vi "Test Timer.vi"() -> ()   [LabVIEW 2012]
doc: "This is an example of how to use the Output Timer class to control the switching behavior fo the CAT system."
uses:
  MSE CAT Controller Demo Source/Type Defs/Output Values.ctl
  MSE CAT Controller Demo Source/Type Defs/AD Settings.ctl
  MSE CAT Controller Demo Source/Type Defs/Output Switches.ctl
  Output Timer/Output Timer.lvclass
  Output Timer/Output Timer.lvclass/Output Timer.ctl
panel:
  out "Numeric":i32
  out "Last Switch":T1 {"[0]" format="%<%H:%M:%S%2u>T"; "[1]" format="%<%H:%M:%S%2u>T"; "[2]" format="%<%H:%M:%S%2u>T"; "[3]" format="%<%H:%M:%S%2u>T"; "[4]" format="%<%H:%M:%S%2u>T"; "[5]" format="%<%H:%M:%S%2u>T"; "[6]" format="%<%H:%M:%S%2u>T"; "[7]" format="%<%H:%M:%S%2u>T"; "[8]" format="%<%H:%M:%S%2u>T"; "[9]" format="%<%H:%M:%S%2u>T"; "[10]" format="%<%H:%M:%S%2u>T"; "[11]" format="%<%H:%M:%S%2u>T"; "[12]" format="%<%H:%M:%S%2u>T"; "[13]" format="%<%H:%M:%S%2u>T"; "[14]" format="%<%H:%M:%S%2u>T"; "[15]" format="%<%H:%M:%S%2u>T"; "[16]" format="%<%H:%M:%S%2u>T"; "[17]" format="%<%H:%M:%S%2u>T"; "[18]" format="%<%H:%M:%S%2u>T"; "[19]" format="%<%H:%M:%S%2u>T"; "[20]" format="%<%H:%M:%S%2u>T"}
  out "Time Stamp":timestamp format="%<%H:%M:%S%2u>T"
  out "Delay S":T2={"Main 1"=inf, "Main 2"=inf, "Recirc  3"=9000.0, "Scrub 4"=8800.0, "O2 5"=9600.0, "Vent 6"=9200.0, "Boost A 7"=3400.0, "Boost A 8"=3400.0, "Recirc  9"=9000.0, "Scrub 10"=8800.0, "Vent 11"=9200.0, "Boost B 12"=1800.0, "Boost B 13"=1800.0, "Recirc 14"=9000.0, "Scrub 15"=8800.0, "Vent 16"=9200.0, "Main 17"=inf, "Boost A 18"=3400.0, "Boost B 19"=1800.0, "Boost F 20"=7000.0, "Vent 2 21"=9200.0}
  out "Final Out":T3
  in  "Final In":T3
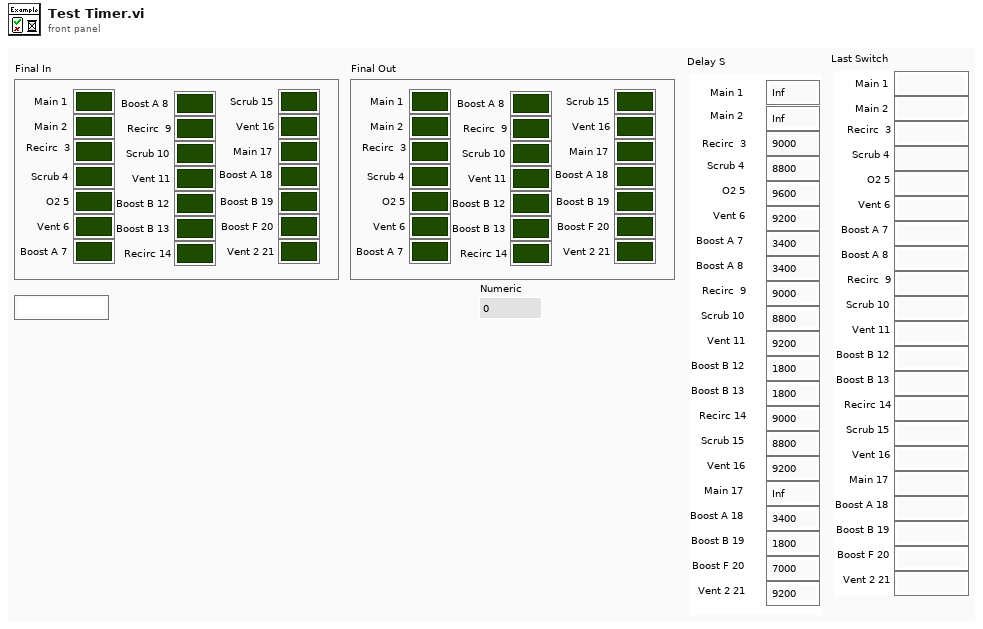
[diagram p1: front panel]
types:
  T1 = cluster{"[0]":timestamp, "[1]":timestamp, "[2]":timestamp, "[3]":timestamp, "[4]":timestamp, "[5]":timestamp, "[6]":timestamp, "[7]":timestamp, "[8]":timestamp, "[9]":timestamp, "[10]":timestamp, "[11]":timestamp, "[12]":timestamp, "[13]":timestamp, "[14]":timestamp, "[15]":timestamp, "[16]":timestamp, "[17]":timestamp, "[18]":timestamp, "[19]":timestamp, "[20]":timestamp}
  T2 = typedef "Output Values.ctl" = cluster{"Main 1":dbl, "Main 2":dbl, "Recirc  3":dbl, "Scrub 4":dbl, "O2 5":dbl, "Vent 6":dbl, "Boost A 7":dbl, "Boost A 8":dbl, "Recirc  9":dbl, "Scrub 10":dbl, "Vent 11":dbl, "Boost B 12":dbl, "Boost B 13":dbl, "Recirc 14":dbl, "Scrub 15":dbl, "Vent 16":dbl, "Main 17":dbl, "Boost A 18":dbl, "Boost B 19":dbl, "Boost F 20":dbl, "Vent 2 21":dbl}
  T3 = cluster{"Main 1":bool, "Main 2":bool, "Recirc  3":bool, "Scrub 4":bool, "O2 5":bool, "Vent 6":bool, "Boost A 7":bool, "Boost A 8":bool, "Recirc  9":bool, "Scrub 10":bool, "Vent 11":bool, "Boost B 12":bool, "Boost B 13":bool, "Recirc 14":bool, "Scrub 15":bool, "Vent 16":bool, "Main 17":bool, "Boost A 18":bool, "Boost B 19":bool, "Boost F 20":bool, "Vent 2 21":bool}
  T4 = typedef "AD Settings.ctl" = cluster{"Set Point Force":T2, "Run A1":T2, "Run A2":T2, "Hold A3":T2, "Hold A4":T2, "High AD Diff ":T5, "Delay S":T2}
  T5 = typedef "Output Switches.ctl" = cluster{"Main 1":bool, "Main 2":bool, "Recirc  3":bool, "Scrub 4":bool, "O2 5":bool, "Vent 6":bool, "Boost A 7":bool, "Boost A 8":bool, "Recirc  9":bool, "Scrub 10":bool, "Vent 11":bool, "Boost B 12":bool, "Boost B 13":bool, "Recirc 14":bool, "Scrub 15":bool, "Vent 16":bool, "Main 17":bool, "Boost A 18":bool, "Boost B 19":bool, "Boost F 20":bool, "Vent 2 21":bool}
  T6 = cluster{"[0]":bool, "[1]":bool, "[2]":bool, "[3]":bool, "[4]":bool, "[5]":bool, "[6]":bool, "[7]":bool, "[8]":bool, "[9]":bool, "[10]":bool, "[11]":bool, "[12]":bool, "[13]":bool, "[14]":bool, "[15]":bool, "[16]":bool, "[17]":bool, "[18]":bool, "[19]":bool, "[20]":bool}
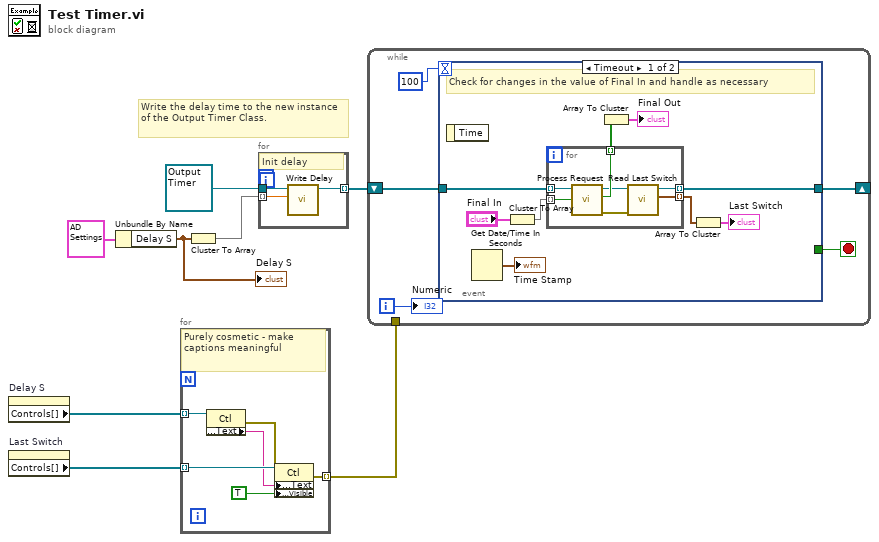
[diagram p0: block diagram]
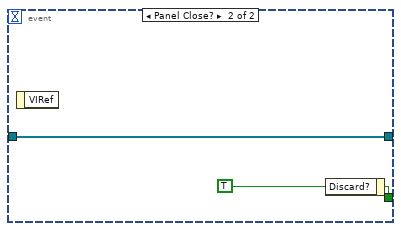
[diagram p2: hidden frame]
diagram:
  # "Write the delay time to the new instance of the Output Timer Class."
  n1 = property on="Delay S" class="Clust (strict)"() -> ("Controls[]"=w3:refnum<vi>[])  [unwired: 2 in, 2 out]
  n2 = property on="Last Switch" class="Clust (strict)"() -> ("Controls[]"=w2:refnum<vi>[])  [unwired: 2 in, 2 out]
  n3 = Unbundle By Name(T4 {"Set Point Force"={"Main 1"=inf, "Main 2"=inf, "Recirc  3"=inf, "Scrub 4"=inf, "O2 5"=inf, "Vent 6"=inf, "Boost A 7"=inf, "Boost A 8"=inf, "Recirc  9"=inf, "Scrub 10"=inf, "Vent 11"=inf, "Boost B 12"=inf, "Boost B 13"=inf, "Recirc 14"=inf, "Scrub 15"=inf, "Vent 16"=inf, "Main 17"=inf, "Boost A 18"=inf, "Boost B 19"=inf, "Boost F 20"=6000.0, "Vent 2 21"=inf}, "Run A1"={"Main 1"=inf, "Main 2"=inf, "Recirc  3"=50.0, "Scrub 4"=inf, "O2 5"=150.0, "Vent 6"=60.0, "Boost A 7"=0.0, "Boost A 8"=0.0, "Recirc  9"=50.0, "Scrub 10"=inf, "Vent 11"=60.0, "Boost B 12"=15.0, "Boost B 13"=15.0, "Recirc 14"=50.0, "Scrub 15"=inf, "Vent 16"=60.0, "Main 17"=inf, "Boost A 18"=0.0, "Boost B 19"=15.0, "Boost F 20"=0.0, "Vent 2 21"=700.0}, "Run A2"={"Main 1"=inf, "Main 2"=inf, "Recirc  3"=-30.0, "Scrub 4"=inf, "O2 5"=80.0, "Vent 6"=15.0, "Boost A 7"=-80.0, "Boost A 8"=-80.0, "Recirc  9"=-30.0, "Scrub 10"=inf, "Vent 11"=15.0, "Boost B 12"=-50.0, "Boost B 13"=-50.0, "Recirc 14"=-30.0, "Scrub 15"=inf, "Vent 16"=15.0, "Main 17"=inf, "Boost A 18"=0.0, "Boost B 19"=-50.0, "Boost F 20"=-80.0, "Vent 2 21"=650.0}, "Hold A3"={"Main 1"=0.0, "Main 2"=0.0, "Recirc  3"=50.0, "Scrub 4"=inf, "O2 5"=150.0, "Vent 6"=60.0, "Boost A 7"=-150.0, "Boost A 8"=-150.0, "Recirc  9"=50.0, "Scrub 10"=inf, "Vent 11"=60.0, "Boost B 12"=-200.0, "Boost B 13"=-200.0, "Recirc 14"=50.0, "Scrub 15"=inf, "Vent 16"=60.0, "Main 17"=0.0, "Boost A 18"=-150.0, "Boost B 19"=-200.0, "Boost F 20"=-200.0, "Vent 2 21"=650.0}, "Hold A4"={"Main 1"=-150.0, "Main 2"=-150.0, "Recirc  3"=-30.0, "Scrub 4"=inf, "O2 5"=80.0, "Vent 6"=15.0, "Boost A 7"=-250.0, "Boost A 8"=-250.0, "Recirc  9"=-30.0, "Scrub 10"=inf, "Vent 11"=15.0, "Boost B 12"=-300.0, "Boost B 13"=-300.0, "Recirc 14"=-30.0, "Scrub 15"=inf, "Vent 16"=15.0, "Main 17"=-150.0, "Boost A 18"=-250.0, "Boost B 19"=-300.0, "Boost F 20"=-300.0, "Vent 2 21"=650.0}, "High AD Diff "={"Main 1"=FALSE, "Main 2"=FALSE, "Recirc  3"=FALSE, "Scrub 4"=TRUE, "O2 5"=FALSE, "Vent 6"=TRUE, "Boost A 7"=FALSE, "Boost A 8"=FALSE, "Recirc  9"=FALSE, "Scrub 10"=TRUE, "Vent 11"=TRUE, "Boost B 12"=FALSE, "Boost B 13"=FALSE, "Recirc 14"=FALSE, "Scrub 15"=TRUE, "Vent 16"=TRUE, "Main 17"=FALSE, "Boost A 18"=FALSE, "Boost B 19"=FALSE, "Boost F 20"=FALSE, "Vent 2 21"=TRUE}, "Delay S"={"Main 1"=30.0, "Main 2"=30.0, "Recirc  3"=1.0, "Scrub 4"=1.0, "O2 5"=1.0, "Vent 6"=1.0, "Boost A 7"=30.0, "Boost A 8"=30.0, "Recirc  9"=1.0, "Scrub 10"=1.0, "Vent 11"=1.0, "Boost B 12"=30.0, "Boost B 13"=30.0, "Recirc 14"=1.0, "Scrub 15"=1.0, "Vent 16"=1.0, "Main 17"=30.0, "Boost A 18"=30.0, "Boost B 19"=30.0, "Boost F 20"=30.0, "Vent 2 21"=1.0}} ("AD Settings")) -> ("Delay S"=w8:T2)
  "Delay S" <- w8
  n4 = for {
    tunnel: w3 -> [w14] mode=indexing
    tunnel: w2 -> [w13] mode=indexing
    tunnel: [w10] -> w1 mode=indexing
    # "Purely cosmetic - make captions meaningful"
    n5 = property class="Ctl"(reference=w14) -> (error out=w11:errorcluster, "Label.Text"=w12:string)  [unwired: 1 in, 1 out]
    n6 = property class="Ctl"(reference=w13, error in=w11, "Caption.Text"=w12, "Caption.Visible"=TRUE) -> (error out=w10:errorcluster)  [unwired: 1 out]
  }
  n7 = Cluster To Array(cluster=w8) -> (array=w7:dbl[])
  n8 = for {
    tunnel: w7 -> [w16] mode=indexing
    tunnel: refnum<class "Output Timer.lvclass"> refnum ("Delay Timer") -> [w17]
    tunnel: [w15] -> w4 mode=indexing
    # "Init delay"
    n9 = call "Write Delay.vi"("Delay"=w16, "Output Timer in"=w17) -> ("Output Timer out"=w15:refnum<class "Output Timer.lvclass">)  [unwired: 8 in, 1 out]
  }
  n10 = while {
    shift-right: [w21] -> _
    shift-left: w4 -> [w22]
    tunnel: w1 -> [_]
    i -> [w18]
    stop <- w19 stop-if-true
    n11 = event shown="[0] Timeout" {
      selector: _ -> [_ _]
      dyn-events: _ -> [_ _]
      timeout: 100 ("Period") -> [_ _]
      tunnel: w22 -> [w29 w39]
      tunnel: [w28 w39] -> w21
      tunnel: [_ w40] -> w19
      event Timeout {
        # "Check for changes in the value of Final In and handle as necessary"
        n12 = event-data() -> ()  [unwired: 1 in, 1 out]
        n13 = Get Date/Time In Seconds() -> (seconds since 1Jan1904=→"Time Stamp":timestamp)
        n14 = Cluster To Array(cluster="Final In") -> (array=w30:bool[])
        n15 = for {
          tunnel: w29 -> [w38] mode=indexing
          tunnel: w30 -> [w37] mode=indexing
          tunnel: [w33] -> w28 mode=indexing
          tunnel: [w36] -> w27 mode=indexing
          tunnel: [w32] -> w24 mode=indexing
          n16 = call "Process Request.vi"("Requested"=w37, "Delay Timer in"=w38) -> ("error out"=w34:errorcluster, "Returned"=w36:bool, "Delay Timer out"=w35:refnum<class "Output Timer.lvclass">)  [unwired: 7 in]
          n17 = call "Read Last Switch.vi"("error in (no error)"=w34, "Output Timer in"=w35) -> ("Last Switch"=w32:timestamp, "Output Timer out"=w33:refnum<class "Output Timer.lvclass">)  [unwired: 7 in, 1 out]
        }
        n18 = Array To Cluster(array=w27) -> (cluster=→"Final Out":T6)
        n19 = Array To Cluster(array=w24) -> (cluster=→"Last Switch":T1)
      }
      event Panel Close? {
        w40 = TRUE ("Discard?")
        n20 = event-data() -> ()  [unwired: 1 in, 1 out]
        n21 = event-data("Discard?"=w40) -> ()  [unwired: 1 in, 1 out]
      }
    }
    "Numeric" <- w18
  }
